vi "ImgCtrl-Get image ctrl.vi"(8 "error in":errorcluster) -> (0 "error out":errorcluster, 3 "Image":T1(plugin-control))   [LabVIEW 2020]
uses:
  <vilib>/vision/Image Controls.llb/IMAQ Image.ctl
  Global variables/gl_Functional Imaging-Global variables.vi
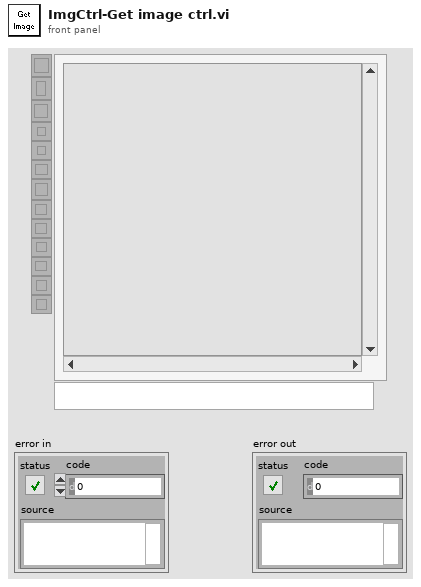
[diagram p1: front panel]
types:
  T1 = typedef "IMAQ Image.ctl" = refnum<image>
  T2 = typedef "Functional Imging UI Refs.ctl" = cluster{"Menu ref":refnum<k9>, "Image control":refnum<vi>, "VI ref":refnum<vi>, "XGrapher":refnum<vi>, "Smoothing":refnum<vi>, "POI Averaging":refnum<vi>, "Normalize":refnum<vi>, "POI data points in each trial":refnum<vi>, "Channel":refnum<vi>, "Experiment data folder path":refnum<vi>, "[ROI vis]":refnum<vi>, "[Groups] visbl":T3, "Group Name":refnum<vi>, "POI index":refnum<vi>, "Trial No.":refnum<vi>, "Intensity Zoom":refnum<vi>, "Trial Cursor Enabled":refnum<vi>, "Number of Trials (ind 1)":refnum<vi>, "Number of Trials (ind 2)":refnum<vi>, "MiniScans Available":refnum<vi>, "POI Available":refnum<vi>, "Defer graph updates":refnum<vi>, "Waveform selector":refnum<vi>, "#of selected POI":refnum<vi>, "#of selected MiniScans":refnum<vi>, "#of selected groups":refnum<vi>, "Max Z-Projection":refnum<vi>, "Z-Plane Selector":refnum<vi>, "Index of miniscan point to visualise":refnum<vi>, "ROI vis. mode":refnum<vi>, "Total # of points":refnum<vi>, "Index of group clicked on":refnum<vi>, "Pane 1":refnum<vi>, "Pane 2":refnum<vi>, "Pane 3":refnum<vi>, "Pane 4":refnum<vi>, "Pane 5":refnum<vi>, "Pane 6":refnum<vi>, "Deselect all ROI":refnum<vi>, "Deselect all groups":refnum<vi>}
  T3 = typedef "Groups array referecne.ctl" = refnum<vi>
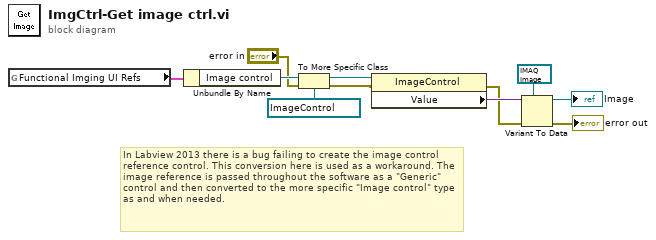
[diagram p0: block diagram]
diagram:
  # "In Labview 2013 there is a bug failing to create the image control reference control. This conversion here is used as a workaround. The image reference is passed throughout the software as a \"Generic\" control and then converted to the more specific \"Image control\" type as and when needed."
  n1 = global read "gl_Functional Imaging-Global variables.vi" "Functional Imging UI Refs"() -> (w6:T2)
  n2 = Unbundle By Name(w6) -> ("Image control"=w5:refnum<vi>)
  n3 = To More Specific Class(target class=refnum<vi> refnum ("Image"), reference=w5, error in="error in") -> (specific class reference=w8:refnum<vi>, error out=w2:errorcluster)
  n4 = property on="Property Node" class="ImageControl"(reference=w8, error in=w2) -> (error out=w4:errorcluster, "Value"=w11:variant)  [unwired: 1 out]
  n5 = Variant To Data(error in=w4, type=T1 refnum ("Image 2"), Variant=w11) -> (data=→"Image":T1, error out=→"error out":errorcluster)
